vi "Convert to RelativePath.vi"(8 "error in (no error)":errorcluster caption="错误输入（无错误）", 11 "VI Path":path) -> (0 "error out":errorcluster caption="错误输出", 3 "RelativePath":string)   [LabVIEW 2016, in "PanelRootNode.lvclass"]
uses:
  PanelRootNode.lvclass
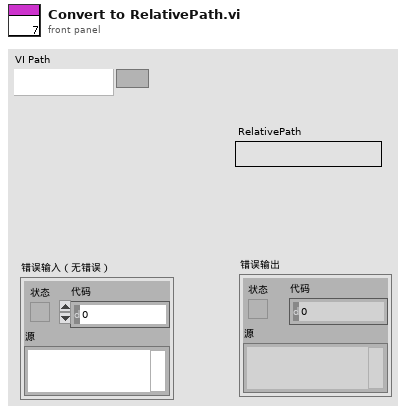
[diagram p1: front panel]
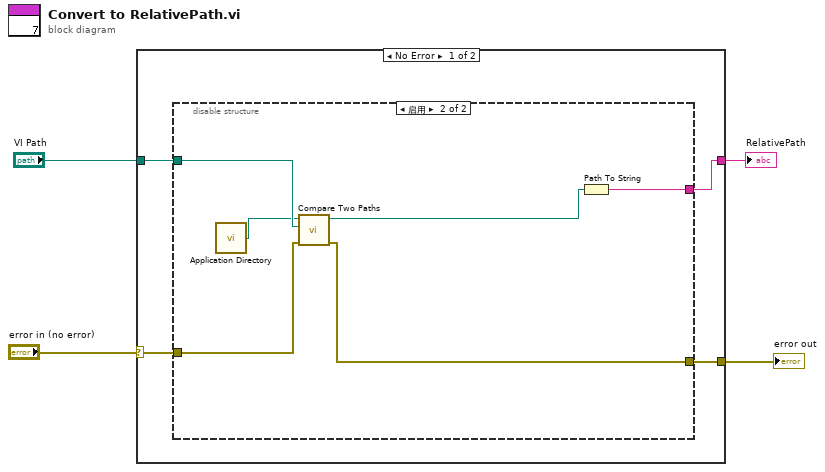
[diagram p0: block diagram]
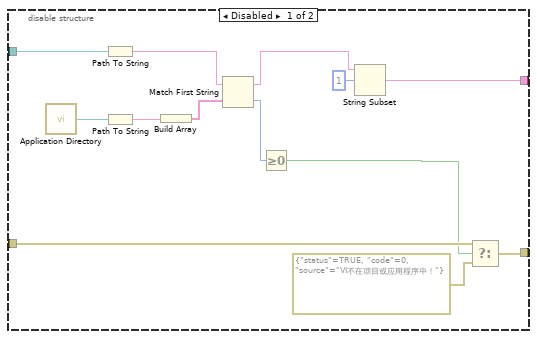
[diagram p2: hidden frame]
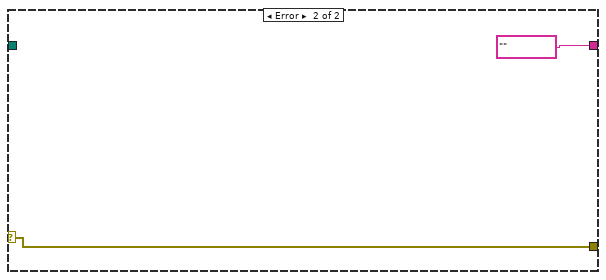
[diagram p3: hidden frame]
diagram:
  n1 = case shown="No Error" "error in (no error)" {
    selector: "error in (no error)" -> [w7 w29]
    tunnel: [w8 w29] -> w4
    tunnel: "VI Path" -> [w6 _]
    tunnel: [w5 ""] -> w1
    frame No Error {
      n2 = disable-structure shown="启用" {
        disable-tunnel: [w20 w23] -> w8
        disable-tunnel: w7 -> [w19 w24]
        disable-tunnel: w6 -> [w18 w27]
        disable-tunnel: [w11 w25] -> w5
        frame Disabled {
          n3 = call <vilib>:"Application Directory.vi"() -> ("Application Directory"=w9:path)
          n4 = Path To String(path=w18) -> (string=w16:string)
          n5 = Path To String(path=w9) -> (string=w15:string)
          n6 = Build Array(w15) -> (w14:string[])
          n7 = Match First String(2:w14, 3:w16) -> (0:w13:i32, 1:w12:string)
          n8 = Greater Or Equal To 0?(x=w13) -> (x >= 0?=w17:bool)
          n9 = String Subset(string=w12, offset (0)=1 ("偏移量(0)")) -> (substring=w11:string)  [unwired: 1 in]
          n10 = Select(t=w19, s=w17, f=errorcluster {"status"=TRUE, "code"=0, "source"="VI不在项目或应用程序中！"}) -> (s? t:f=w20:errorcluster)
        }
        frame Enabled {
          n11 = call <vilib>:"Application Directory.vi"() -> ("Application Directory"=w22:path)
          n12 = call <vilib>:"Compare Two Paths.vi"("error in (no error)"=w24, "Path 2"=w27, "Path 1"=w22) -> ("error out"=w23:errorcluster, "Relative Path from 1 to 2"=w26:path)  [unwired: 5 in, 2 out]
          n13 = Path To String(path=w26) -> (string=w25:string)
        }
      }
    }
    frame Error {
    }
  }
  "error out" <- w4
  "RelativePath" <- w1
